vi "MockFAILC.vi"(11 "MockFAILCSettings":T1={"ModbusRxDataFIFO"="ModbusSubnetARxDataFIFO", "ModbusTxDataFIFO"="ModbusSubnetATxDataFIFO", "BufferUpdateFIFO"="MockFAILC1Command", "Code17Memory"="MockFAILC1Code17", "Code18Memory"="MockFAILC1Code18", "Code65Memory"="MockFAILC1Code65", "Code72Memory"="MockFAILC1Code72", "Code74Memory"="MockFAILC1Code74", "Code75Memory"="MockFAILC1Code75", "Code76Memory"="MockFAILC1Code76", "Code80Memory"="MockFAILC1Code80", "Code110Memory"="MockFAILC1Code110", "Code120Memory"="MockFAILC1Code120", "Code121Memory"="MockFAILC1Code121", "CRCDataFIFO"="MockFAILC1CRCDataFIFO", "CRCCalculateFIFO"="MockFAILC1CRCCalculateFIFO", "CRCFIFO"="MockFAILC1CRCFIFO", "Code119Memory"="MockFAILC1Code119"}) -> ()   [LabVIEW 2016, in "FPGAMockFAILC.lvlib"]
uses:
  FPGAMockFAILC.lvlib
  DataTypes/MockFAILCSettings.ctl
  Common_FPGA_Modbus/DataTypes/ModbusCRCSettings.ctl
  Common_FPGA_Modbus/FPGAModbus.lvlib
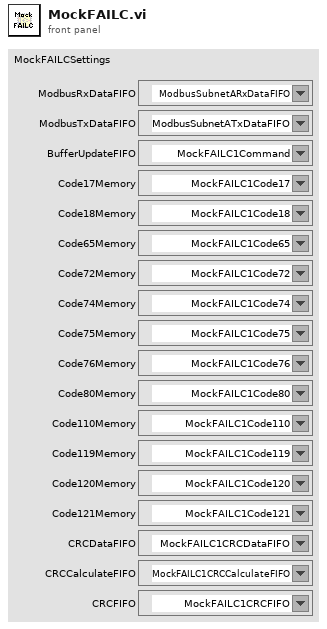
[diagram p1: front panel]
types:
  T1 = typedef "FPGAMockFAILC.lvlib/MockFAILCSettings.ctl" = cluster{"ModbusRxDataFIFO":refnum<k21>, "ModbusTxDataFIFO":refnum<k21>, "BufferUpdateFIFO":refnum<k21>, "Code17Memory":refnum<k21>, "Code18Memory":refnum<k21>, "Code65Memory":refnum<k21>, "Code72Memory":refnum<k21>, "Code74Memory":refnum<k21>, "Code75Memory":refnum<k21>, "Code76Memory":refnum<k21>, "Code80Memory":refnum<k21>, "Code110Memory":refnum<k21>, "Code120Memory":refnum<k21>, "Code121Memory":refnum<k21>, "CRCDataFIFO":refnum<k21>, "CRCCalculateFIFO":refnum<k21>, "CRCFIFO":refnum<k21>, "Code119Memory":refnum<k21>}
  T2 = typedef "FPGAModbus.lvlib/ModbusCRCSettings.ctl" = cluster{"DataFIFO":refnum<k21>, "CalculateFIFO":refnum<k21>, "OutputFIFO":refnum<k21>}
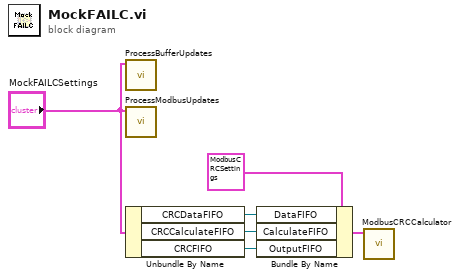
[diagram p0: block diagram]
diagram:
  n1 = call "ProcessBufferUpdates.vi"("MockFAILCSettings"="MockFAILCSettings") -> ()  [unwired: 11 in]
  n2 = call "ProcessModbusUpdates.vi"("MockFAILCSettings"="MockFAILCSettings") -> ()  [unwired: 11 in]
  n3 = Unbundle By Name("MockFAILCSettings") -> ("CRCDataFIFO"=w4:refnum<k21>, "CRCCalculateFIFO"=w3:refnum<k21>, "CRCFIFO"=w2:refnum<k21>)
  n4 = Bundle By Name(cluster=T2 {"DataFIFO"="MockHPILCCRCDataFIFO", "CalculateFIFO"="MockHPILCCRCCalculateFIFO", "OutputFIFO"="MockHPILCCRCFIFO"} ("ModbusCRCSettings"), "DataFIFO"=w4, "CalculateFIFO"=w3, "OutputFIFO"=w2) -> (w5:T2)
  n5 = call "ModbusCRCCalculator.vi"("ModbusCRCSettings"=w5) -> ()  [unwired: 11 in]
